vi "PH_Beckhoff.set Analog Outputs Defaults.vi"(1 "Service IDs":i32[](array[numeric]), 2 "Sca Type":u32[](array[numeric]), 3 "Analog Output Tag Names":string[](array[string])) -> (0 "Analog Outputs":T2)   [LabVIEW 2014, in "PH_Beckhoff.lvlib"]
uses:
  PH_Beckhoff.lvlib
  PH_Beckhoff.Analog Outputs.ctl
  PH_Beckhoff.Scaling Type.ctl
panel:
  in  "Analog Output Value":T1={"Name"="", "Value"=0, "Quality"=FALSE, "Wanted Value"=0, "Service ID"=-1, "Sca Type"=0}
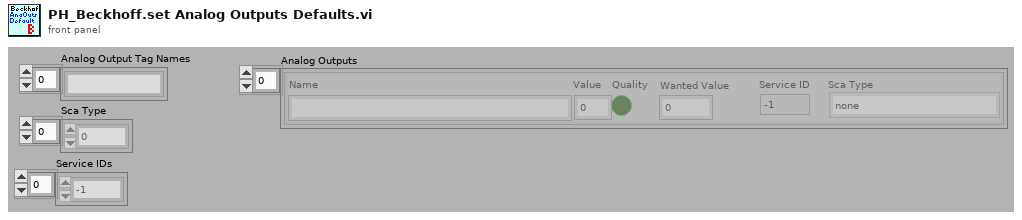
[diagram p1: front panel]
types:
  T1 = cluster{"Name":string, "Value":u32, "Quality":bool, "Wanted Value":u32, "Service ID":i32, "Sca Type":u32}
  T2 = typedef "PH_Beckhoff.lvlib/PH_Beckhoff.Analog Outputs.ctl" = cluster{"Name":string, "Value":u32, "Quality":bool, "Wanted Value":u32, "Service ID":i32, "Sca Type":T3}[]
  T3 = typedef "PH_Beckhoff.lvlib/PH_Beckhoff.Scaling Type.ctl" = enum16{"none", "0 ... 15 Bit -> 0 ... 5", "0 ... 15 Bit -> 0 ... 10", "0 ... 15 Bit -> 0 ... 25", "0 ... 15 Bit -> 4 ... 20", "0 ... 15 Bit -> 0 ... 1", "0 ... 15 Bit -> 0 ... 20000", "0 ... 15 Bit -> 0 ... 24000"}
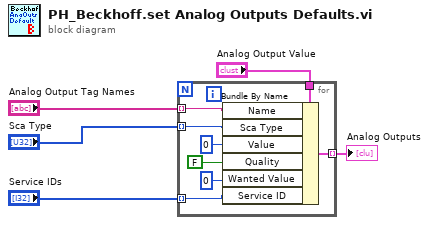
[diagram p0: block diagram]
diagram:
  n1 = for {
    tunnel: "Analog Output Value" -> [w13]
    tunnel: [w12] -> w4 mode=indexing
    tunnel: "Analog Output Tag Names" -> [w11] mode=indexing
    tunnel: "Sca Type" -> [w10] mode=indexing
    tunnel: "Service IDs" -> [w6] mode=indexing
    n2 = Bundle By Name(cluster=w13, "Name"=w11, "Sca Type"=w10, "Value"=u32 0, "Quality"=FALSE, "Wanted Value"=u32 0, "Service ID"=w6) -> (w12:T1)
  }
  "Analog Outputs" <- w4
